vi "Accelerometer one direction.vi"() -> ()   [LabVIEW 2014]
uses:
  <vilib>/Simulation/Scripting/Companion Diagram/SimConfigNode/SimParams.ctl
  <vilib>/Simulation/Scripting/Companion Diagram/SimConfigNode/_simSolvers.ctl
  <vilib>/Simulation/Implementation/Shared/SIMSCR Execution Mode.ctl
  <vilib>/Simulation/Param Hierarchy/Typedefs/SIMPH Param Control Actions.ctl
  <vilib>/Simulation/Implementation/Shared/SIM limit type.ctl
  <vilib>/Simulation/Implementation/Shared/NILVSim_ParamChanged.vi
  <vilib>/Simulation/Implementation/Shared/NILVSIM_BeginStep.vi
  <vilib>/Simulation/DataSources/Implementation/NILVSim Step.llb/SIM Step (scalar).vi
  <vilib>/Simulation/DataSources/Implementation/NILVSim Ramp.llb/SIM Ramp (scalar).vi
  <vilib>/Simulation/ContinuousLinear/Implementation/NILVSim Integrator new.llb/SIM Integrator distributor (scalar).vi
  <vilib>/Simulation/SignalArithmetic/Implementation/NILVSim Gain.llb/SIM Gain (scalar).vi
  <vilib>/Simulation/Utility/Implementation/NILVSim Memory.llb/NILVSim Memory (core).vi
  <vilib>/Simulation/ContinuousLinear/Implementation/NILVSim Integrator new.llb/SIM Integrator collector (scalar).vi
  <vilib>/Simulation/SignalDisplay/Implementation/NILVSim Time Waveform.llb/SIM Time Waveform (vector).vi
  <vilib>/Simulation/Implementation/Shared/NILVSim_Manager.vi
  <vilib>/Utility/error.llb/Clear Errors.vi
  <vilib>/Simulation/Implementation/Shared/NILVSim_FinalizeModel.vi
  <vilib>/Simulation/Implementation/Shared/SIM Unbundle Sim Info.vi
  <vilib>/Simulation/Implementation/Shared/NILVSim_Initialize.vi
  <vilib>/Simulation/Utility/Implementation/NILVSim Get Time and IsAcceptedStep.vi
  <vilib>/Simulation/Implementation/Shared/SIMSH Read Queue.vi
  <vilib>/Simulation/Implementation/Shared/NILVSim_GetModelError.vi
  <vilib>/Simulation/Implementation/Shared/SIM Bundle Sim Info.vi
  <vilib>/Simulation/Scripting/Companion Diagram/SimConfigNode/SimDog.xnode
  <vilib>/Simulation/Implementation/XNodeFramework/SimXNode/SimX.xnode
  <vilib>/Simulation/ContinuousLinear/Implementation/NILVSim Integrator new.llb/SIM Integrator (scalar).vi
  <vilib>/Simulation/Implementation/Shared/NI_SIM_Implementation.lvlib
panel:
  in  "R initial output":dbl
  in  "R Start time":dbl=0.5
  in  "R Slope":dbl=1.0
  in  "final Value":dbl=0.0001
  in  "Step time":dbl=0.5
  in  "R":dbl=300.0
  in  "C":dbl=0.01
  in  "A":dbl=1.0
  in  "K":dbl=0.001
  in  "b":dbl=10.0
  in  "Kq 2":dbl=10.0
  in  "Kq":dbl=10.0
  in  "m":dbl=0.4
  out "Waveform Chart":waveform(dbl)[](graph)=[{"t0"=timestamp(1 s since 1904-01-01), "dt"=1.0, "Y"=[0.5]}, {"t0"=timestamp(1 s since 1904-01-01), "dt"=1.0, "Y"=[0.0011396753898964128]}]
  # "Title: Accelerometer one direction, Bond Graph\nAuthor: Jad Saud \nDate: 2019.10.03\nVersion: v1.0"
  # "RAMP RESPONS"
  # "Step Respons (disconnected)"
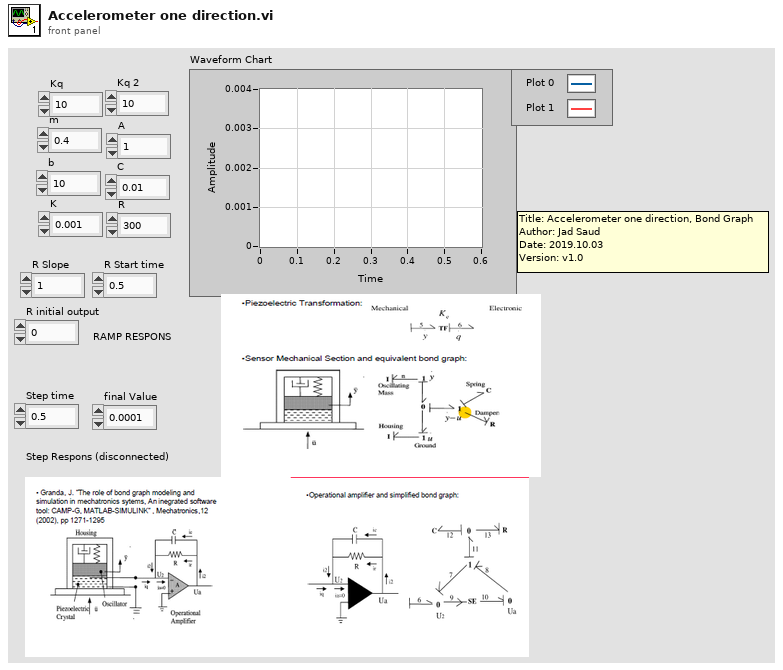
[diagram p1: front panel]
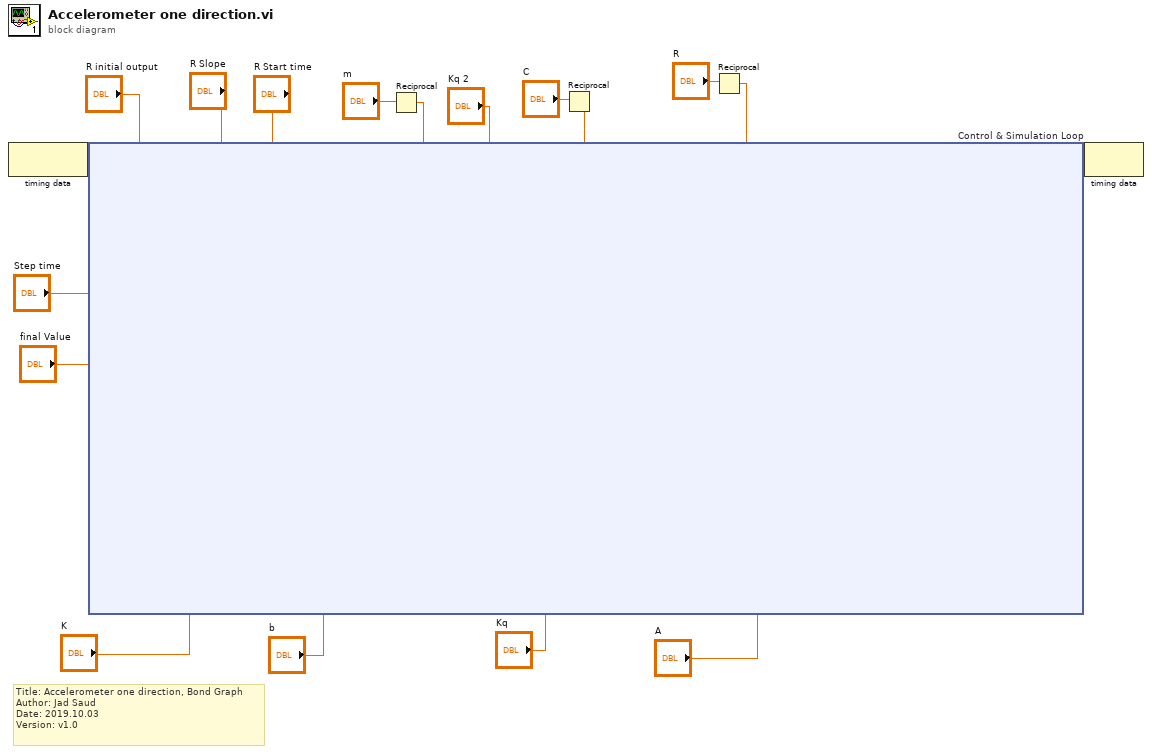
[diagram p0: block diagram]
diagram:
  # "Title: Accelerometer one direction, Bond Graph\nAuthor: Jad Saud \nDate: 2019.10.03\nVersion: v1.0"
  n1 = node-c288() -> (w18:variant)  [unwired: 1 in]
  n2 = Reciprocal(x="m") -> (1/x=w15:dbl)
  n3 = Reciprocal(x="C") -> (1/x=w10:dbl)
  n4 = Reciprocal(x="R") -> (1/x=w8:dbl)
  n5 = node-c254 "Control & Simulation Loop"(w18, w15, "Kq", "Kq 2", "K", "b", "A", w10, w8, "Step time", "final Value", "R Slope", "R Start time", "R initial output") -> (w17:variant)
  n6 = node-c288(w17) -> ()  [unwired: 1 out]
